vi "Find Child Unified Actor.vi"(7 "Actor in":refnum<class "Actor.lvclass">, 10 "Unified Actor Alias":string) -> (1 "Found":bool, 2 "Child Unified Actor":T1)   [LabVIEW 2020, in "jettl.lvlib"]
uses:
  jettl.lvlib
  Message/Message.lvclass
  Actor/Actor.lvclass
  MessageSet.ctl
  Messages.ctl
  ActorRelation.ctl
  MessageMetadata.ctl
  Message.ctl
  Actor.ctl
  ActorLifetime.ctl
  ActorType.ctl
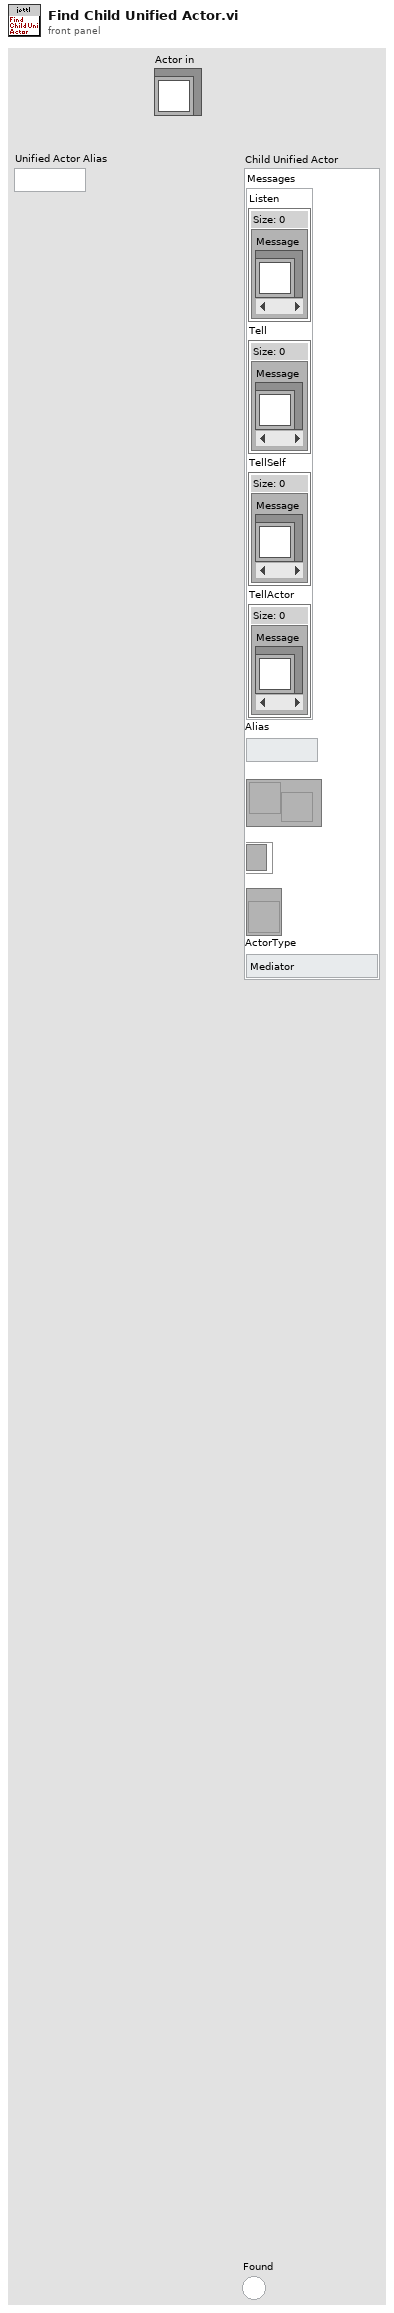
[diagram p1: front panel]
types:
  T1 = typedef "jettl.lvlib/Actor.ctl" = cluster{"Messages":T2, "Alias":string, "Transport":refnum<user-event>, "Address":refnum<event-registration>, "VIRef":refnum<vi>, "ActorType":T4}
  T2 = typedef "jettl.lvlib/Messages.ctl" = cluster{"Listen":T3, "Tell":T3, "TellSelf":T3, "TellActor":T3}
  T3 = typedef "jettl.lvlib/MessageSet.ctl" = set{refnum<class "Message.lvclass">}
  T4 = typedef "jettl.lvlib/ActorType.ctl" = enum16{"Mediator", "Component"}
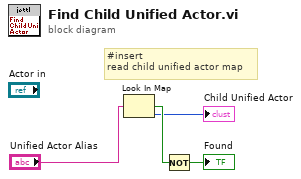
[diagram p0: block diagram]
diagram:
  # "#insert\nread child unified actor map"
  n1 = Look In Map(key="Unified Actor Alias") -> (key not found?=w3:bool, value=→"Child Unified Actor":i32)  [unwired: 2 in]
  n2 = Not(x=w3) -> (.not. x?=→"Found":bool)
